vi "Weather Station UI.vi"() -> ()   [LabVIEW 2012]
doc: "This is the main VI in the Weather Station Project. It contains the user interface for a temperature warning system. Temperature is retrieved every half second; data is logged when a warning has occurred."
uses:
  Supporting Files/Weather Station States.ctl
  Supporting Files/Weather Data.ctl
  Instance           2 26Saved   Weather Station UI .vi
panel:
  out "Warning":string
  in  "Lower Limit":dbl=20.0
  in  "Upper Limit":dbl=30.0
  in  "Stop Button":bool
  out "Temperature History":dbl(graph)
  # "Temperature Ranges (C)"
  # "Freeze"
  # "Heat \nStroke"
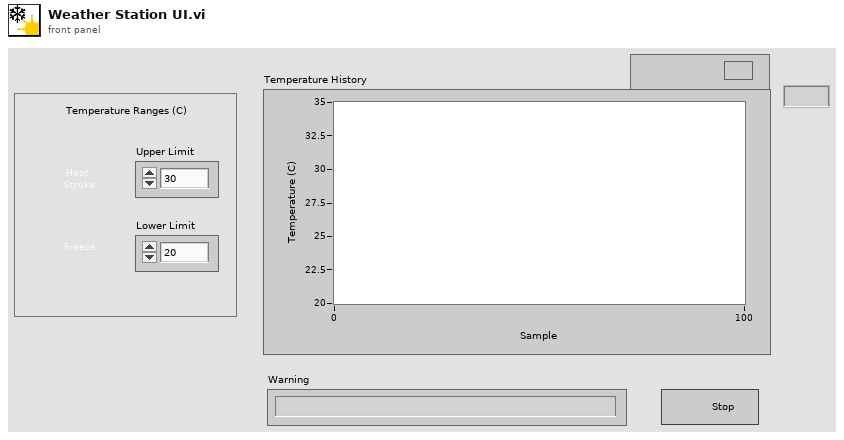
[diagram p1: front panel]
types:
  T1 = enum16{"open", "replace", "create", "open or create", "replace or create", "replace or create with confirmation"}
  T2 = typedef "Weather Data.ctl" = cluster{"Current Temperature":dbl, "Max Temperature":dbl, "Min Temperature":dbl, "Temperature Warning?":bool, "Temperature Warning Text":string}
  T3 = typedef "Weather Station States.ctl" = enum16{"Acquisition", "Range Check", "Analysis", "Data Log", "Time Check"}
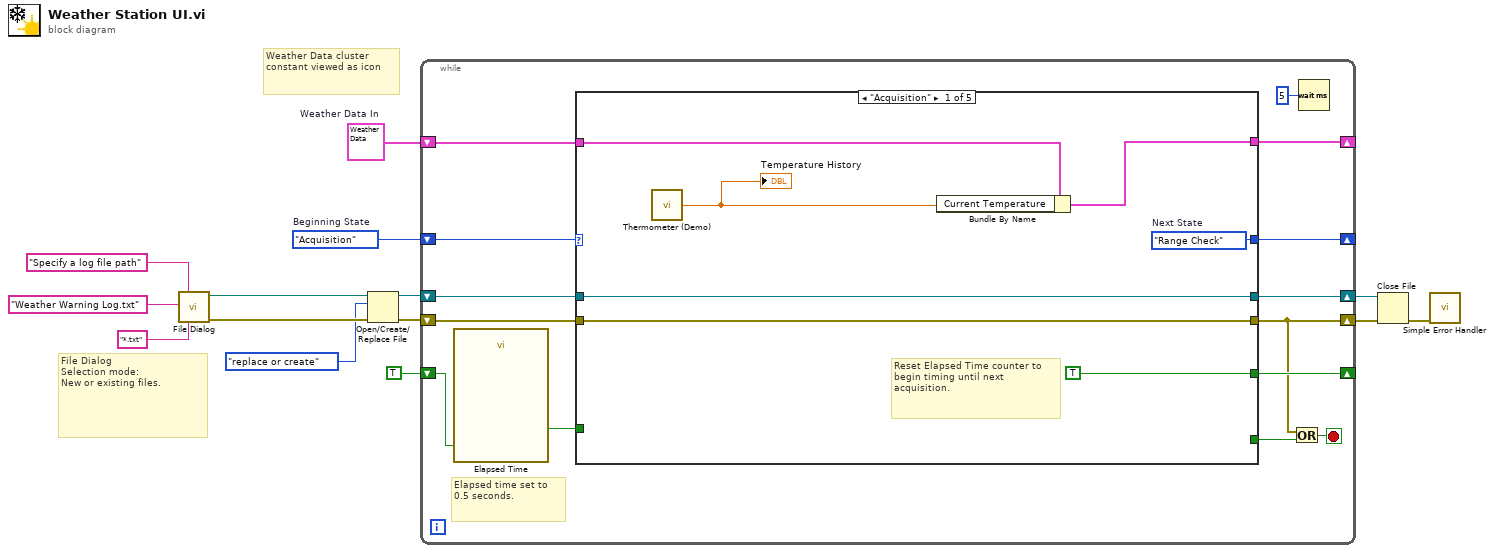
[diagram p0: block diagram]
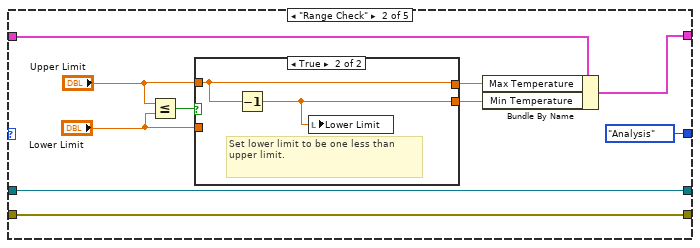
[diagram p2: hidden frame]
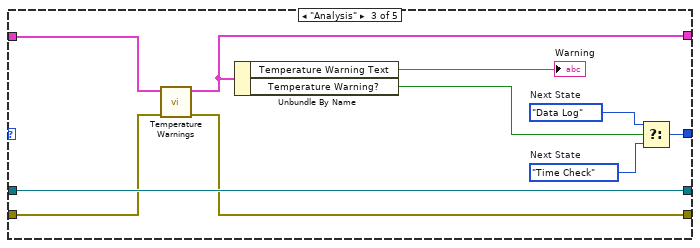
[diagram p4: hidden frame]
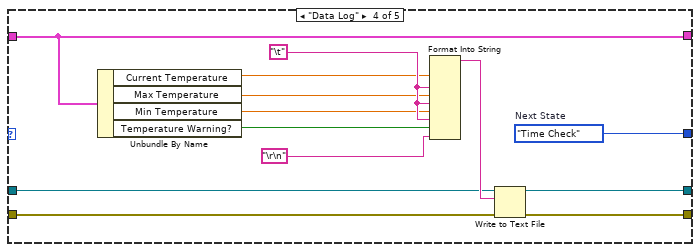
[diagram p5: hidden frame]
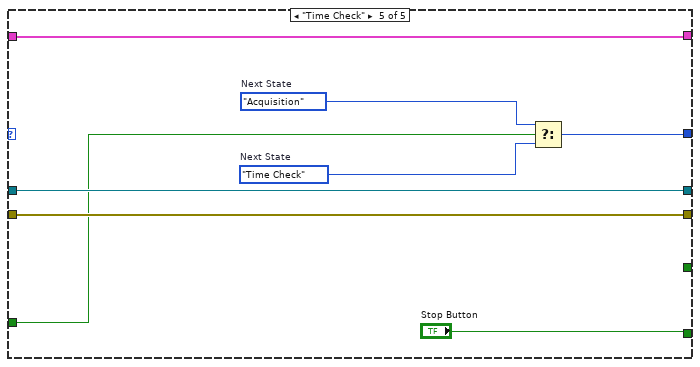
[diagram p6: hidden frame]
diagram:
  w7 = T2 {"Current Temperature"=0.0, "Max Temperature"=0.0, "Min Temperature"=0.0, "Temperature Warning?"=FALSE, "Temperature Warning Text"="No Warning"}  # Weather Data In
  w14 = Weather_Station_States."Acquisition"  # Beginning State
  # "File Dialog\nSelection mode:\nNew or existing files."
  # "Weather Data cluster\nconstant viewed as icon"
  n1 = call "File Dialog"("prompt"="Specify a log file path", "default name"="Weather Warning Log.txt", "pattern (all files)"="*.txt" ("pattern label")) -> ("selected path"=w6:path, "error out"=w3:errorcluster)  [unwired: 9 in, 2 out]
  n2 = Open/Create/Replace File(file path (use dialog)=w6, error in=w3, operation (0:open)=T1."replace or create") -> (refnum out=w9:refnum<file>, error out=w8:errorcluster)  [unwired: 3 in, 1 out]
  n3 = while {
    shift-right: [w27] -> _
    shift-left: w14 -> [w28]
    shift-right: [w15] -> w13
    shift-left: w8 -> [w26]
    shift-right: [w16] -> _
    shift-left: w7 -> [w23]
    shift-right: [w24] -> w12
    shift-left: w9 -> [w22]
    shift-right: [w17] -> _
    shift-left: TRUE ("stop") -> [w19]
    stop <- w25 stop-if-true
    # "Elapsed time set to\n0.5 seconds."
    n4 = call "Elapsed Time"("Reset"=w19) -> ("Time has Elapsed"=w18:bool)  [unwired: 11 in, 7 out]
    n5 = case shown="\"Acquisition\"" w28 {
      tunnel: [w35 Weather_Station_States."Analysis" ("Next State") w53 w72 w73] -> w27
      tunnel: [w30 w45 w57 w70 w79] -> w15
      tunnel: w26 -> [w30 w45 w58 w71 w79]
      tunnel: [w34 w44 w59 w69 w80] -> w24
      tunnel: [w31 w41 w52 w60 w78] -> w16
      tunnel: w23 -> [w32 w42 w50 w60 w78]
      tunnel: w22 -> [w34 w44 w59 w67 w80]
      tunnel: [_ _ _ _ "Stop Button"] -> w21
      tunnel: w18 -> [_ _ _ _ w74]
      tunnel: [TRUE ("stop") _ _ _ _] -> w17
      frame "Acquisition" {
        w35 = Weather_Station_States."Range Check"  # Next State
        # "Reset Elapsed Time counter to begin timing until next acquisition."
        n6 = call "Thermometer (Demo).vi"() -> ("Temperature Value"=w29:dbl)  [unwired: 1 in]
        "Temperature History" <- w29
        n7 = Bundle By Name(cluster=w32, "Current Temperature"=w29) -> (w31:T2)
      }
      frame "Range Check" {
        n8 = Less Or Equal?(x="Upper Limit", y="Lower Limit") -> (x <= y?=w40:bool)
        n9 = case shown="True" w40 {
          tunnel: "Upper Limit" -> [w47 w49]
          tunnel: "Lower Limit" -> [w46 _]
          tunnel: [w47 w49] -> w37
          tunnel: [w46 w48] -> w36
          frame False {
          }
          frame True {
            # "Set lower limit to be one less than\nupper limit."
            n10 = Decrement(x=w49) -> (x-1=w48:dbl)
            n11 = local write "Lower Limit"(w48) -> ()
          }
        }
        n12 = Bundle By Name(cluster=w42, "Max Temperature"=w37, "Min Temperature"=w36) -> (w41:T2)
      }
      frame "Analysis" {
        w55 = Weather_Station_States."Data Log"  # Next State
        w54 = Weather_Station_States."Time Check"  # Next State
        n13 = call "Temperature Warnings.vi"("Error In"=w58, "Weather Data In"=w50) -> ("Error Out"=w57:errorcluster, "Weather Data Out"=w52:T2)  [unwired: 8 in]
        n14 = Unbundle By Name(w52) -> ("Temperature Warning Text"=→"Warning":string, "Temperature Warning?"=w56:bool)
        n15 = Select(t=w55, s=w56, f=w54) -> (s? t:f=w53:T3)
      }
      frame "Data Log" {
        w72 = Weather_Station_States."Time Check"  # Next State
        w66 = "\t"
        n16 = Unbundle By Name(w60) -> ("Current Temperature"=w65:dbl, "Max Temperature"=w64:dbl, "Min Temperature"=w63:dbl, "Temperature Warning?"=w62:bool)
        n17 = Format Into String(w65, w66, w64, w66, w63, w66, w62, "\r\n") -> (resulting string=w68:string)  [unwired: 3 in, 1 out]
        n18 = Write to Text File(file (use dialog)=w67, text=w68, error in=w71) -> (refnum out=w69:refnum<file>, error out=w70:errorcluster)  [unwired: 1 in, 1 out]
      }
      frame "Time Check" {
        w76 = Weather_Station_States."Time Check"  # Next State
        w75 = Weather_Station_States."Acquisition"  # Next State
        n19 = Select(t=w75, s=w74, f=w76) -> (s? t:f=w73:T3)
      }
    }
    n20 = Or(x=w15, y=w21) -> (x .or. y?=w25:bool)
    n21 = Wait (ms)(milliseconds to wait=u32 5 ("y")) -> ()  [unwired: 1 out]
  }
  n22 = Close File(refnum=w12, error in=w13) -> (error out=w11:errorcluster)  [unwired: 1 out]
  n23 = call <vilib>:"Simple Error Handler.vi"("error in (no error)"=w11) -> ()  [unwired: 4 in, 5 out]
